vi "TEST - Get Strings from Enum.vi"(8 "error in (no error)":errorcluster) -> (0 "error out":errorcluster, 2 "pass":bool)   [LabVIEW 2020]
uses:
  source/library/oglib_lvdata.lvlib
panel:
  out "Failures":T1(array[cluster])
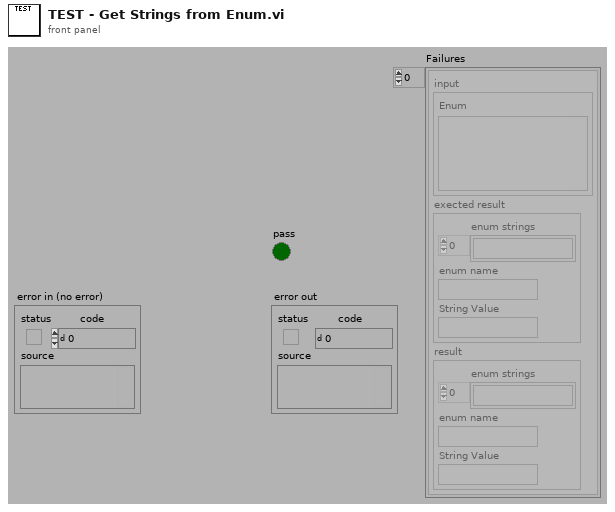
[diagram p1: front panel]
types:
  T1 = cluster{"input":cluster{"Enum":variant}, "exected result":cluster{"enum strings":string[], "enum name":string, "String Value":string}, "result":cluster{"enum strings":string[], "enum name":string, "String Value":string}}[]
  T2 = cluster{"input":cluster{"Enum":variant}, "exected result":cluster{"enum strings":string[], "enum name":string, "String Value":string}, "result":cluster{"enum strings":string[], "enum name":string, "String Value":string}}
  T3 = cluster{"enum strings":string[], "enum name":string, "String Value":string}
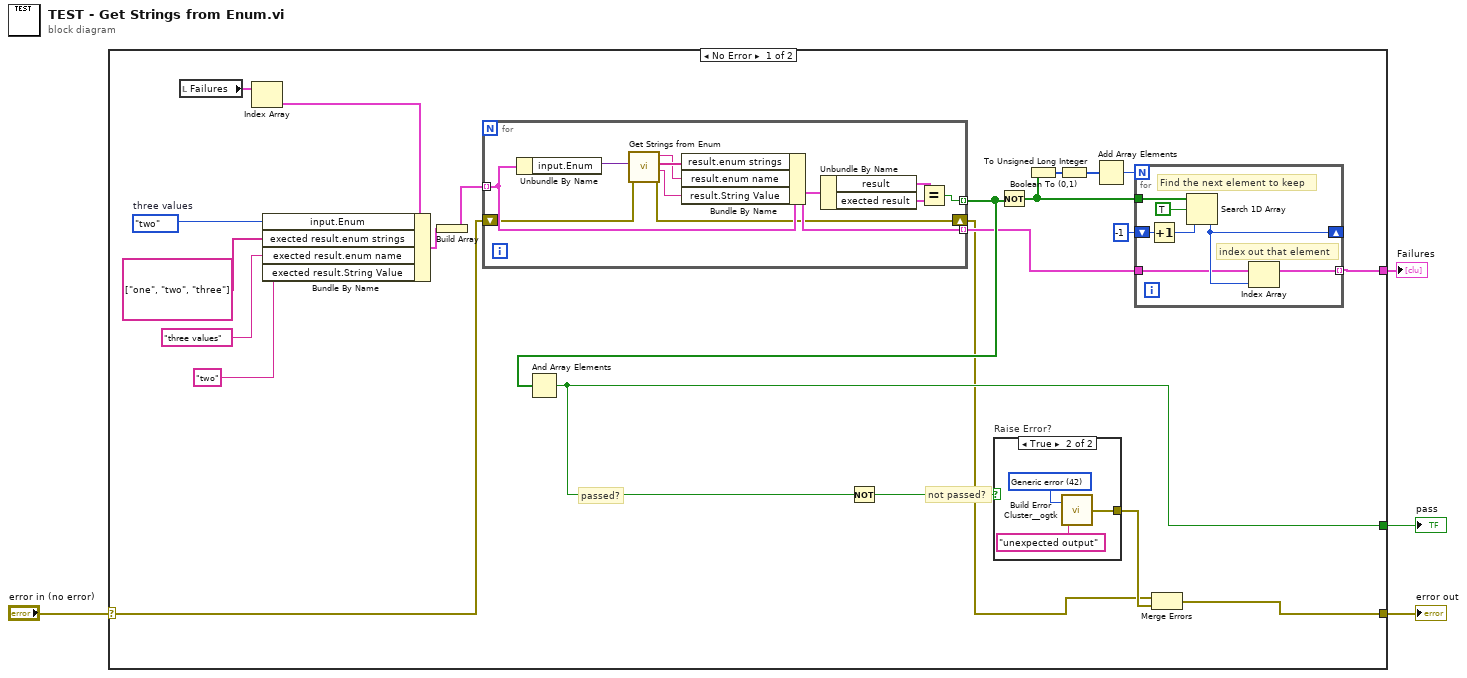
[diagram p0: block diagram]
diagram:
  n1 = case shown="No Error" "error in (no error)" {
    selector: "error in (no error)" -> [w12 w48]
    tunnel: [w23 _] -> w4
    tunnel: [w26 w48] -> w2
    tunnel: [w15 _] -> w1
    frame No Error {
      w8 = enum16{"one", "two", "three"}."two"  # three values
      # "not passed?"
      # "passed?"
      n2 = local read "Failures"() -> (w10:T1)
      n3 = Index Array(array=w10) -> (element=w9:T2)  [unwired: 1 in]
      n4 = Bundle By Name(cluster=w9, "input.Enum"=w8, "exected result.enum strings"=string[] ["one", "two", "three"], "exected result.enum name"="three values", "exected result.String Value"="two") -> (w14:T2)
      n5 = Build Array(w14) -> (w13:T1)
      n6 = for {
        tunnel: w13 -> [w43] mode=indexing
        tunnel: [w44] -> w17 mode=indexing
        tunnel: [w42] -> w16 mode=indexing
        shift-right: [w39] -> w11
        shift-left: w12 -> [w38]
        n7 = Unbundle By Name(w43) -> ("input.Enum"=w37:variant)
        n8 = call "Get Strings from Enum.vi"("error in (no error)"=w38, "Enum"=w37) -> ("error out"=w39:errorcluster, "String Value"=w34:string, "Enum Strings"=w36:string[], "Enum Name"=w35:string)  [unwired: 6 in]
        n9 = Bundle By Name(cluster=w43, "result.enum strings"=w36, "result.enum name"=w35, "result.String Value"=w34) -> (w42:T2)
        n10 = Unbundle By Name(w42) -> ("result"=w41:T3, "exected result"=w40:T3)
        n11 = Equal?(x=w41, y=w40) -> (x = y?=w44:bool)
      }
      n12 = And Array Elements(Boolean array=w17) -> (logical AND=w23:bool)
      n13 = Not(x=w23) -> (.not. x?=w24:bool)
      n14 = case "Raise Error?" shown="True" w24 {
        tunnel: [_ w45] -> w25
        frame False {
        }
        frame True {
          w46 = 42 items=["No error", "Argument error", "Memory is full", "Out of zone", "End of file", "File already open", "Generic file I/O error", "File not found", "File permission error", "Disk is full", "Duplicate path", "Too many files open", "System feature not enabled", "Resource file not found", "Cannot add resource", "Resource not found", "Image not found", "Image memory error", "Pen does not exist", "Config type invalid", "Config token not found", "Config parse error", "Config memory error", "Bad external code format", "Bad external code offset", "External code not present", "Null window", "Destroy window error", "Null menu", "Print aborted", "Bad print record", "Print driver error", "Windows error during printing", "Memory error during printing", "Print dialog error", "Generic print error", "Invalid device refnum", "Device not found", "Device parameter error", "Device unit error", "Cannot open device", "Device call aborted", "Generic error", "Cancelled by user", "Object ID too low", "Object ID too high", "Object not in heap", "Unknown heap", "Unknown object (invalid DefProc)", "Unknown object (DefProc not in table)", "Message out of range", "Invalid (null) method", "Unknown message", "Manager call not supported", "Bad address", "Network operation in progress", "Network operation timed out", "Connection is busy", "Network attribute not supported", "Network error", "Address in use", "System out of memory", "Connection aborted", "Connection refused", "Not connected", "Already connected", "Connection closed", "Initialization error (interapplication manager)", "Bad occurrence", "Wait on unbound occurrence handler", "Occurrence queue overflow", "Datalog type conflict", "Unused", "Unrecognized type (interapplication manager)", "Memory corrupt", "Failed to make temporary DLL", "Old CIN version", "Drag socket not found", "Failed to load drop-object", "Failed to register OLE object", "Failed to release OLE object", "Format specifier type mismatch", "Unknown format specifier", "Too few format specifiers", "Too many format specifiers", "Scan failed", "Newer CIN version", "Error converting to variant", "Runtime menu error", "Password tampered", "Variant attribute not found", "Incompatible variant data type", "Event data is not available", "Event Store is not present", "Occurrence is not found", "Event Queue is not created", "Event info is not available", "Refnum passed is NULL", "Error retrieving Class GUID", "Error retrieving CoClass GUID", "Error retrieving TypeLib GUID.", "Bad built application magic bytes.", "Specific driver is different from the specific driver associated with the Logical Name.", "There is no session opened to the class driver.", "Max Error", "MAX - Error with config objects", "MAX - Error loading configuration", "MAX - Group not supported"]
          n15 = call <userlib>:"Build Error Cluster__ogtk.vi"("String to Prepend to source (\"\")"="unexpected output" ("String to Prepend to source (\"\")"), "code"=w46) -> ("error out"=w45:errorcluster)
        }
      }
      n16 = Not(x=w17) -> (.not. x?=w19:bool[])
      n17 = Boolean To (0,1)(Boolean=w19) -> (0, 1=w20:i16[])
      n18 = To Unsigned Long Integer(number=w20) -> (unsigned 32bit integer=w18:u32[])
      n19 = Add Array Elements(numeric array=w18) -> (sum=w21:u32)
      n20 = for {
        N: w21 -> [_]
        tunnel: w16 -> [w29]
        tunnel: w19 -> [w33]
        shift-right: [w30] -> _
        shift-left: -1 ("start index (0)") -> [w31]
        tunnel: [w28] -> w15 mode=indexing
        # "index out that element"
        # "Find the next element to keep"
        n21 = Increment(x=w31) -> (x+1=w27:i32)
        n22 = Search 1D Array(1D array=w33, element=TRUE, start index (0)=w27) -> (index of element=w30:i32)
        n23 = Index Array(array=w29, index=w30) -> (element=w28:T2)
      }
      n24 = Merge Errors(w11, w25) -> (w26:errorcluster)
    }
    frame Error {
    }
  }
  "pass" <- w4
  "error out" <- w2
  "Failures" <- w1
